vi "1.1)Comandos trigger (SubVI).vi"(3 "?":bool, 4 "Opciones de Trigger":enum32{"Flanco", "Video", "Pulso"}(tab)) -> (20 "Comando a Enviar":string)   [LabVIEW 2014]
panel:
  out "concatenated string":string
  in  "Holdoff":dbl(knob) scale=5e-07..10.0
  in  "Nivel":dbl(knob) scale=-20.0..20.0
  in  "Mode":u16(ring) items=["Auto", "Normal"]
  in  "Estado":bool
  in  "Forzar":bool
  in  "Frecuencia":bool
  out "Comando final Trigger":string
  out "Tipo de trigger":string
  in  "Canal":u16(ring) items=["Canal 1", "Canal 2"]
  in  "Slope":u16(ring) items=["Fall", "Rise"]
  in  "Acoplamiento":u16(ring) items=["AC", "DC", "Sin altas frecuencias DC", "Sin bajas frecuencias AC", "Baja sensibilidad DC"]
  in  "Sync":u16(ring) items=["Field", "Line", "Odd", "Even", "LineNum"]
  in  "Polarity":u16(ring) items=["Inverted", "Normal"]
  in  "Lines":dbl(knob) scale=0.0..525.0
  in  "Standard":u16(ring) items=["NTSC", "PAL"]
  in  "Canal":u16(ring) items=["Canal 1", "Canal 2"]
  in  "Width":dbl(knob) scale=3.3e-08..10.0
  in  "When":u16(ring) items=["Equal", "NotEqual", "Inside", "Outside"]
  in  "Polarity":u16(ring) items=["Positivo", "Negativo"]
  in  "Ancho":u16(ring) items=["Polarity", "When", "Width"]
  in  "Canal":u16(ring) items=["Canal 1", "Canal 2"]
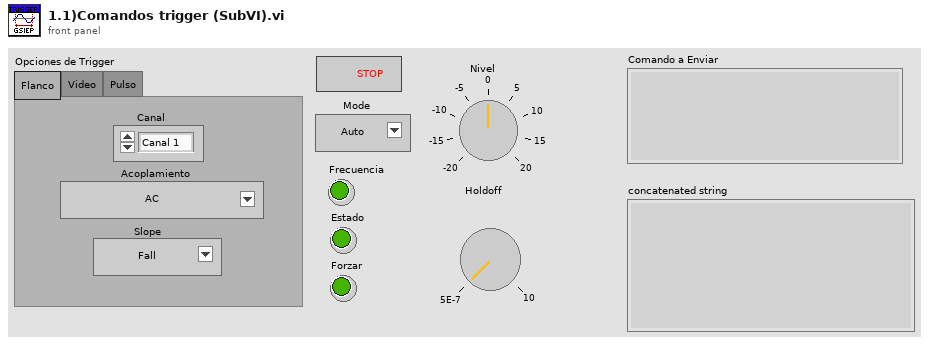
[diagram p1: front panel]
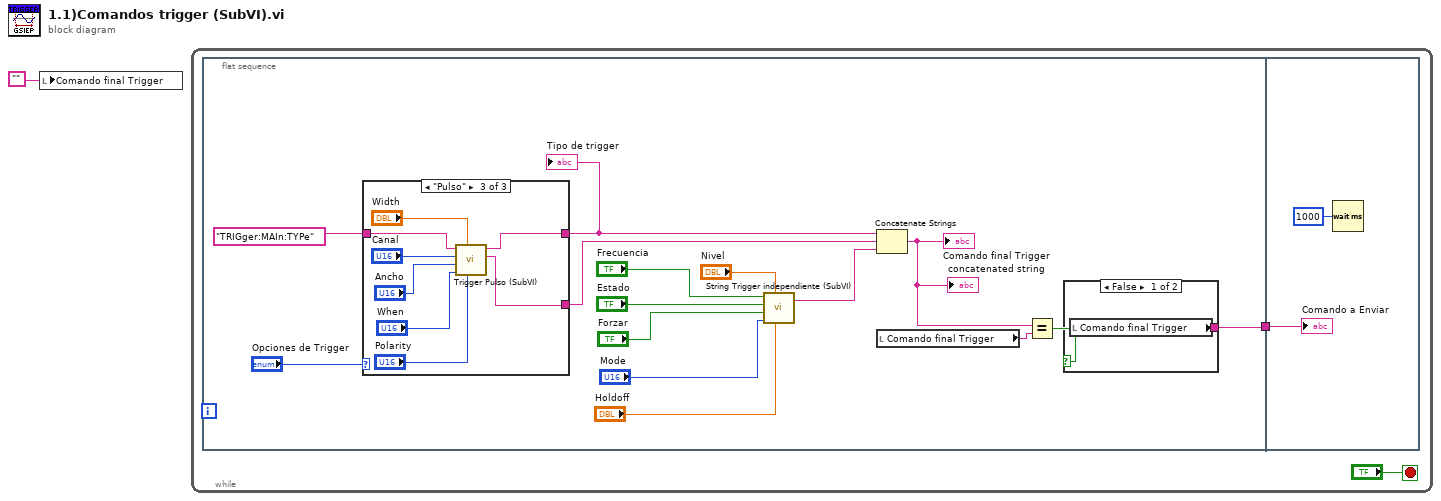
[diagram p0: block diagram]
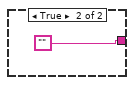
[diagram p2: hidden frame]
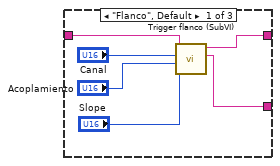
[diagram p3: hidden frame]
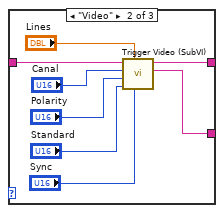
[diagram p4: hidden frame]
diagram:
  n1 = local write "Comando final Trigger"("") -> ()
  n2 = while {
    stop <- "?" stop-if-true
    n3 = flat-sequence {
      tunnel: [w13] -> w3
      tunnel: w3 -> [w44]
      frame #0 {
        n4 = case shown="\"Pulso\"" "Opciones de Trigger" {
          tunnel: "TRIGger:MAIn:TYPe" -> [w25 w31 w42]
          tunnel: [w26 w33 w41] -> w18
          tunnel: [w21 w32 w40] -> w17
          frame "Flanco", Default {
            n5 = call "Trigger flanco (SubVI).vi"("Slope"="Slope", "Acoplamiento"="Acoplamiento", "Canal"="Canal", "String de Entrada"=w25) -> ("String de Salida"=w21:string, "String de tipo"=w26:string)  [unwired: 6 in]
          }
          frame "Video" {
            n6 = call "Trigger Video (SubVI).vi"("Sync"="Sync", "Lines"="Lines", "Standard"="Standard", "Polarity"="Polarity", "Canal"="Canal", "String de Entrada"=w31) -> ("String de Salida"=w32:string, "String de Tipo"=w33:string)  [unwired: 4 in]
          }
          frame "Pulso" {
            n7 = call "Trigger Pulso (SubVI).vi"("Polarity"="Polarity", "Width"="Width", "When"="When", "Ancho"="Ancho", "Canal"="Canal", "String de Entrada"=w42) -> ("String de Salida"=w40:string, "String de Tipo"=w41:string)  [unwired: 4 in]
          }
        }
        "Tipo de trigger" <- w18
        n8 = call "String Trigger independiente (SubVI).vi"("Holdoff"="Holdoff", "Nivel"="Nivel", "Mode"="Mode", "Force"="Forzar", "State"="Estado", "Frecuency"="Frecuencia") -> ("String trigges independiente"=w4:string)  [unwired: 1 in]
        n9 = Concatenate Strings(w18, w17, w4) -> (w16:string)
        "Comando final Trigger" <- w16
        "concatenated string" <- w16
        n10 = local read "Comando final Trigger"() -> (w15:string)
        n11 = Equal?(x=w16, y=w15) -> (x = y?=w14:bool)
        n12 = case shown="False" w14 {
          tunnel: [w19 ""] -> w13
          frame False {
            n13 = local read "Comando final Trigger"() -> (w19:string)
          }
          frame True {
          }
        }
      }
      frame #1 {
        n14 = Wait (ms)(milliseconds to wait=u32 1000) -> ()  [unwired: 1 out]
        "Comando a Enviar" <- w44
      }
    }
  }
